vi "matlab_TI2_moveToXYZ.vi"(8 "error in":errorcluster, 9 "zset":dbl, 10 "yset":dbl, 11 "xset":dbl) -> (0 "error out":errorcluster, 2 "XYZpos":cluster{dbl, dbl, dbl})   [LabVIEW 2018]
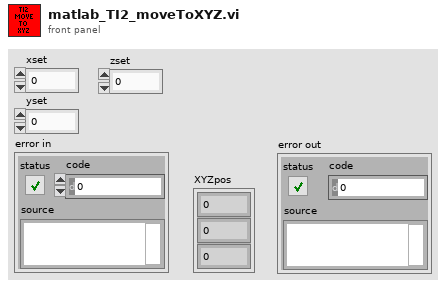
[diagram p1: front panel]
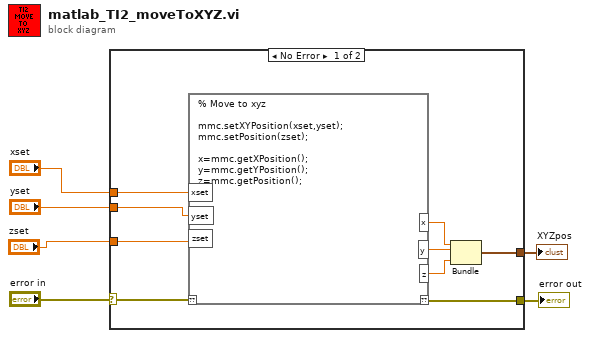
[diagram p0: block diagram]
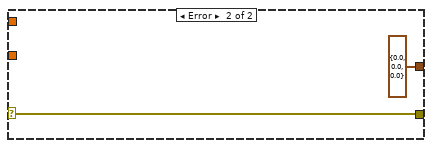
[diagram p2: hidden frame]
diagram:
  n1 = case shown="No Error" "error in" {
    selector: "error in" -> [w15 w17]
    tunnel: [w14 w17] -> w5
    tunnel: "xset" -> [w13 _]
    tunnel: "yset" -> [w12 _]
    tunnel: [w8 cluster{dbl, dbl, dbl} {0.0, 0.0, 0.0}] -> w4
    tunnel: "zset" -> [w7 _]
    frame No Error {
      n2 = script code="% Move to xyz\n\nmmc.setXYPosition(xset,yset);\nmmc.setPosition(zset);\n\nx=mmc.getXPosition();\ny=mmc.getYPosition();\nz=mmc.getPosition();"("??"=w15, "xset"=w13, "yset"=w12, "zset"=w7) -> ("??"=w14:errorcluster, "x"=w10:dbl, "y"=w11:dbl, "z"=w9:dbl)
      n3 = Bundle(w10, w11, w9) -> (w8:cluster{dbl, dbl, dbl})  [unwired: 1 in]
    }
    frame Error {
    }
  }
  "error out" <- w5
  "XYZpos" <- w4
